vi "GetCallingProcessCloneName.vi"(10 "call chain":string[](array[string])) -> (2 "Process Clone":string)   [LabVIEW 2021, in "smo.lvlib" / "SMO.lvclass"]
uses:
  SMO.lvclass
  SMO.lvclass/SMO.ctl
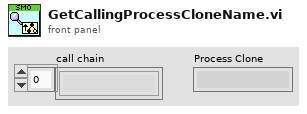
[diagram p1: front panel]
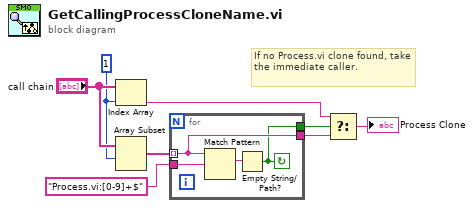
[diagram p0: block diagram]
diagram:
  w7 = 1 ("Index")
  # "If no Process.vi clone found, take the immediate caller."
  n1 = Index Array(array="call chain", index=w7) -> (element=w1:string)
  n2 = Array Subset(array="call chain", index=w7) -> (w5:string[])  [unwired: 1 in]
  n3 = for {
    tunnel: w5 -> [w10] mode=indexing
    tunnel: "Process.vi:[0-9]+$" ("regular expression") -> [w12]
    tunnel: [w10] -> w3
    tunnel: [w9] -> w2
    stop <- w9 continue-if-true
    n4 = Match Pattern(string=w10, regular expression=w12) -> (match substring=w11:string)  [unwired: 1 in, 3 out]
    n5 = Empty String/Path?(string/path=w11) -> (empty?=w9:bool)
  }
  n6 = Select(t=w1, s=w2, f=w3) -> (s? t:f=→"Process Clone":string)
